vi "IsBoardFull.vi"(1 "Board":i32[][](array[numeric])) -> (0 "full":bool)   [LabVIEW 2025]
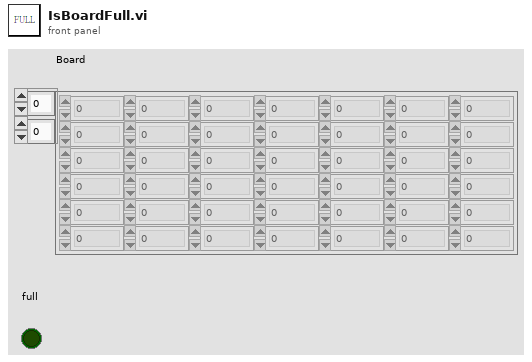
[diagram p1: front panel]
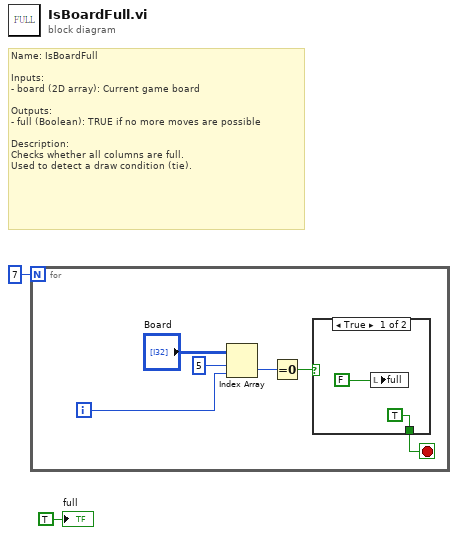
[diagram p0: block diagram]
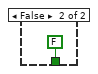
[diagram p2: hidden frame]
diagram:
  # "Name: IsBoardFull\n\nInputs:\n- board (2D array): Current game board\n\nOutputs:\n- full (Boolean): TRUE if no more moves are possible\n\nDescription:\nChecks whether all columns are full.\nUsed to detect a draw condition (tie)."
  n1 = for {
    N: 7 -> [_]
    i -> [w5]
    stop <- w3 stop-if-true
    n2 = Index Array(array="Board", index (row)=5, index (col)=w5) -> (element=w7:i32)
    n3 = Equal To 0?(x=w7) -> (x = 0?=w4:bool)
    n4 = case shown="True" w4 {
      tunnel: [TRUE FALSE] -> w3
      frame True {
        n5 = local write "full"(FALSE ("Boolean")) -> ()
      }
      frame False {
      }
    }
  }
  "full" <- TRUE ("Boolean")
